vi "calculateSetpoints.vi"(8 "error in (no error)":errorcluster, 10 "Sensor Data":T4 {"Robot Heading" format="%05.1f"; "Wind Direction" format="%05.1f"}, 11 "Desired Location":T5) -> (0 "error out":errorcluster, 3 "Setpoints":T1)   [LabVIEW 2011]
uses:
  2 Typedefs/UTM Location.ctl
  2 Typedefs/sensorData.ctl
  2 Typedefs/heading.ctl
  2 Typedefs/setpoints to boat.ctl
  2 Typedefs/sail setpt.ctl
  2 Typedefs/rudder angle.ctl
  2 Typedefs/apparent wind direction.ctl
  2 Typedefs/Velocity.ctl
panel:
  in  "Small RC LUT":dbl[][](array[numeric])=[[0.0, 0.0, 0.0, 0.0, 0.0, 0.0, 0.0, 0.0, 0.0, 0.0, 0.055, 0.111, 0.166, 0.222, 0.277, 0.333, 0.388, 0.444, 0.5, 0.5278, 0.5556, 0.5833, 0.6111, 0.6389, 0.6667, 0.6944, 0.7222, 0.75, 0.7778, 0.8056, 0.8333, 0.8611, 0.8889, 0.9167, 0.9444, 0.9722, 1.0], [1.0, 0.9722, 0.9444, 0.9167, 0.8889, 0.8611, 0.8333, 0.8056, 0.7778, 0.75, 0.7222, 0.6944, 0.6667, 0.6389, 0.6111, 0.5833, 0.5556, 0.5278, 0.5, 0.4444, 0.3889, 0.3333, 0.2778, 0.2222, 0.1667, 0.1111, 0.0556, 0.0, 0.0, 0.0, 0.0, 0.0, 0.0, 0.0, 0.0, 0.0, 0.0]]
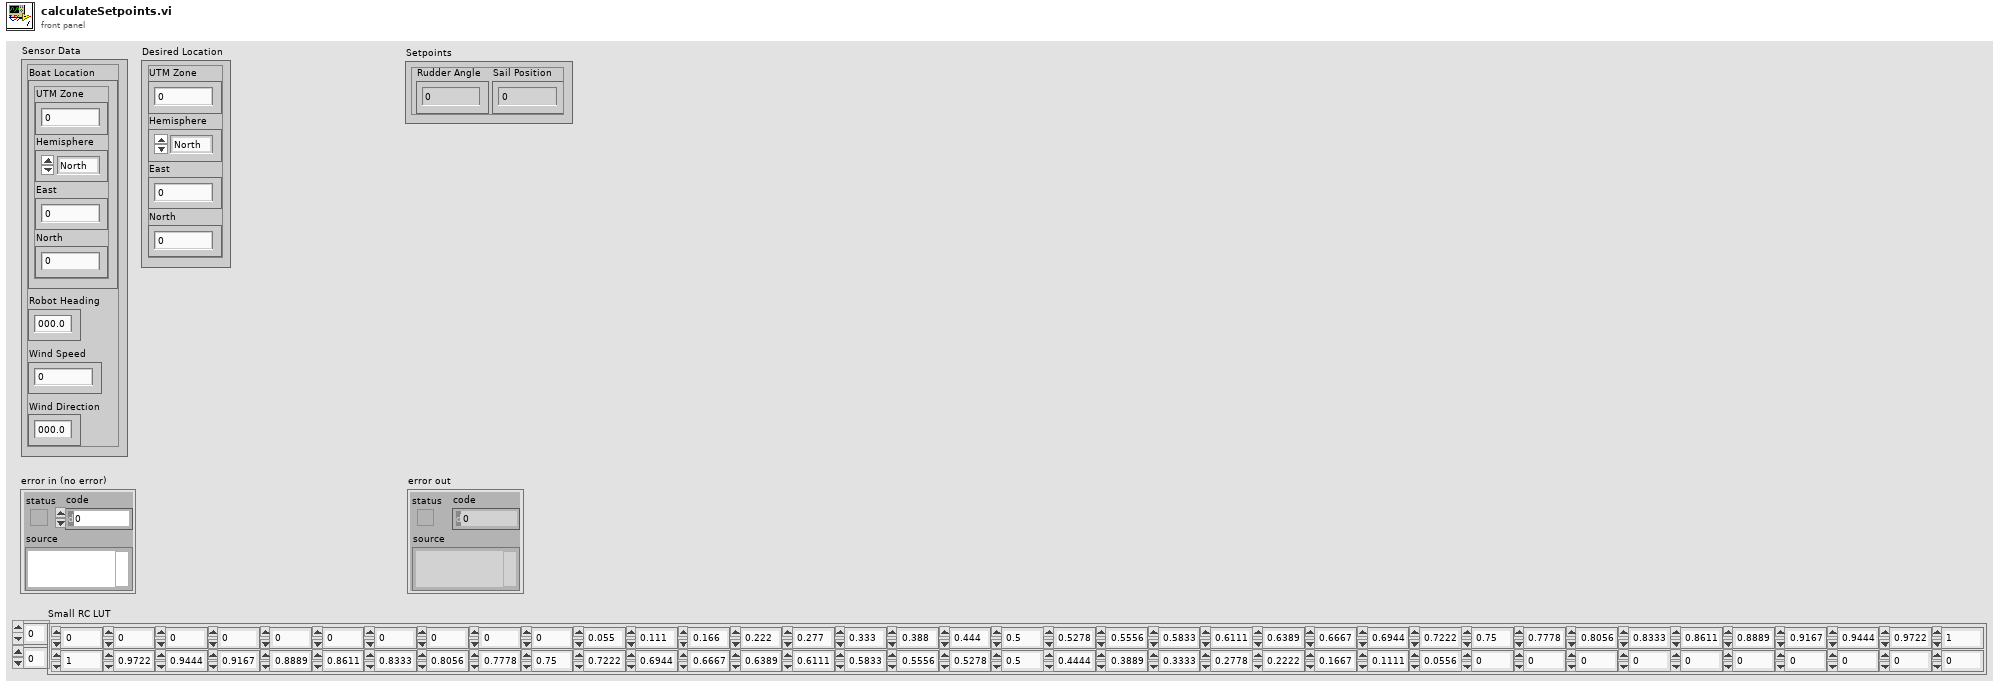
[diagram p1: front panel]
types:
  T1 = typedef "setpoints to boat.ctl" = cluster{"Sail Position":T2, "Rudder Angle":T3}
  T2 = typedef "sail setpt.ctl" = dbl
  T3 = typedef "rudder angle.ctl" = dbl
  T4 = typedef "sensorData.ctl" = cluster{"Boat Location":T5, "Robot Heading ":T6, "Wind Speed":dbl, "Wind Direction":T6}
  T5 = typedef "UTM Location.ctl" = cluster{"UTM Zone":dbl, "Hemisphere":enum16{"North", "South"}, "East":dbl, "North":dbl}
  T6 = typedef "heading.ctl" = dbl
  T7 = typedef "apparent wind direction.ctl" = dbl
  T8 = typedef "Velocity.ctl" = cluster{"East":dbl, "North":dbl}
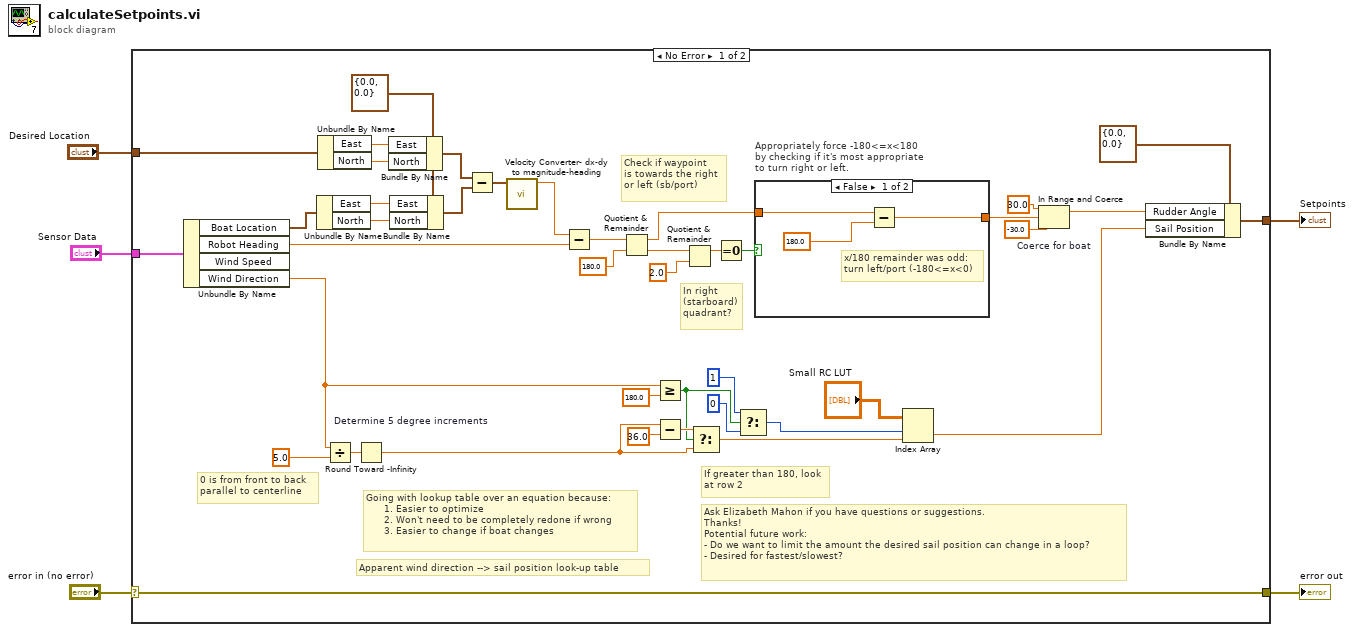
[diagram p0: block diagram]
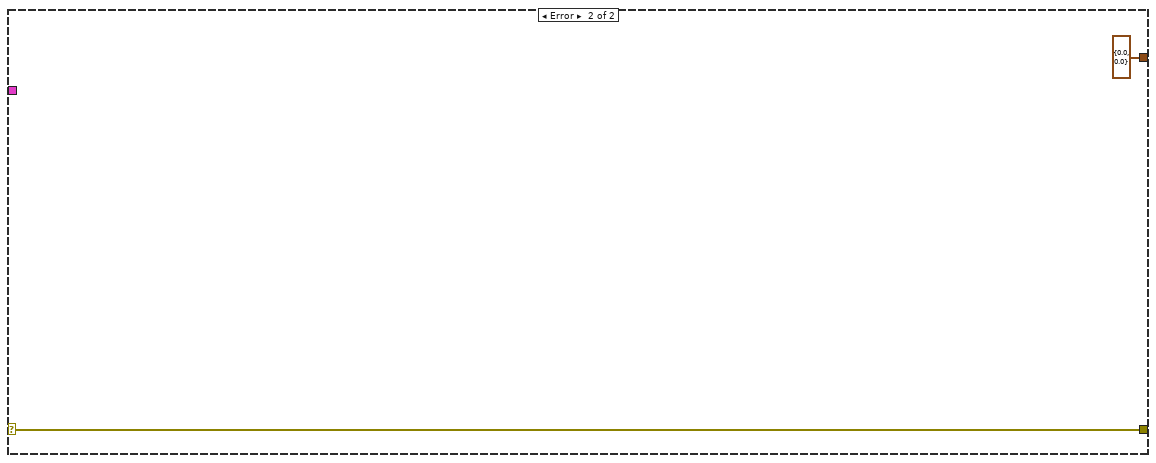
[diagram p3: hidden frame]
diagram:
  n1 = case shown="No Error" "error in (no error)" {
    selector: "error in (no error)" -> [w46 w52]
    tunnel: [w46 w52] -> w4
    tunnel: "Sensor Data" -> [w45 _]
    tunnel: "Desired Location" -> [w23 _]
    tunnel: [w20 T1 {"Sail Position"=0.0, "Rudder Angle"=0.0} ("Setpoints")] -> w1
    frame No Error {
      w44 = T8 {"East"=0.0, "North"=0.0} ("Vector In")
      # "Ask Elizabeth Mahon if you have questions or suggestions.\nThanks!\nPotential future work:\n- Do we want to limit the amount the desired sail position can change in a loop?\n- Desired for fastest/slowest?"
      # "If greater than 180, look\nat row 2"
      # "Apparent wind direction --> sail position look-up table"
      # "0 is from front to back\nparallel to centerline"
      # "Going with lookup table over an equation because:\n      1. Easier to optimize\n      2. Won't need to be completely redone if wrong\n      3. Easier to change if boat changes"
      # "Check if waypoint\nis towards the right\nor left (sb/port)"
      # "In right\n(starboard)\nquadrant?"
      n2 = Unbundle By Name(w45) -> ("Boat Location"=w34:T5, "Robot Heading"=w35:T6, "Wind Direction"=w8:T6)  [unwired: 1 out]
      n3 = Unbundle By Name(w34) -> ("East"=w41:dbl, "North"=w40:dbl)
      n4 = Unbundle By Name(w23) -> ("East"=w43:dbl, "North"=w42:dbl)
      n5 = Divide(x=w8, y=T7 5.0) -> (x/y=w10:T6)
      n6 = Round Toward -Infinity "Determine 5 degree increments"(1:w10) -> (0:w18:T6)
      n7 = Bundle By Name(cluster=w44, "East"=w43, "North"=w42) -> (w39:T8)
      n8 = Bundle By Name(cluster=w44, "East"=w41, "North"=w40) -> (w38:T8)
      n9 = Subtract(x=w39, y=w38) -> (x-y=w37:T8)
      n10 = call "Velocity Converter- dx-dy to magnitude-heading.vi"("Vector In"=w37) -> ("Heading Out"=w36:T6)  [unwired: 9 in, 1 out]
      n11 = Subtract(x=w36, y=w35) -> (x-y=w24:T6)
      n12 = Quotient & Remainder ("shift to -180<x<180")(x=w24, y=T6 180.0) -> (x-y*floor(x/y)=w32:T6, floor(x/y)=w28:T6)
      n13 = Greater Or Equal?(x=w8, y=T7 180.0) -> (x >= y?=w15:bool)
      n14 = Subtract(x=w18, y=T7 36.0) -> (x-y=w17:T6)
      n15 = Quotient & Remainder ("shift to -180<x<180")(x=w28, y=T6 2.0) -> (x-y*floor(x/y)=w30:T6)  [unwired: 1 out]
      n16 = Select(t=w17, s=w15, f=w18) -> (s? t:f=w19:T6)
      n17 = Equal To 0?(x=w30) -> (x = 0?=w31:bool)
      n18 = Select(t=1, s=w15, f=0) -> (s? t:f=w14:i32)
      n19 = case "Appropriately force -180<=x<180\nby checking if it's most appropriate\nto turn right or left." shown="False" w31 {
        tunnel: w32 -> [w48 w50]
        tunnel: [w47 w50] -> w33
        frame False {
          # "x/180 remainder was odd:\nturn left/port (-180<=x<0)"
          n20 = Subtract(x=w48, y=T6 180.0) -> (x-y=w47:T6)
        }
        frame True {
          # "x/180 remainder was\neven: turn right/sb\n(0<=x<180)"
        }
      }
      n21 = Index Array(array="Small RC LUT", index (row)=w14, index (col)=w19) -> (element=w6:dbl)
      n22 = In Range and Coerce "Coerce for boat"(upper limit=T6 30.0, x=w33, lower limit=T6 -30.0) -> (coerced(x)=w21:T6)  [unwired: 1 out]
      n23 = Bundle By Name(cluster=T1 {"Sail Position"=0.0, "Rudder Angle"=0.0} ("Setpoints"), "Rudder Angle"=w21, "Sail Position"=w6) -> (w20:T1)
    }
    frame Error {
    }
  }
  "error out" <- w4
  "Setpoints" <- w1
